vi "Edit Dialog.vi"(11 "Content":string) -> (2 "OK?":bool, 3 "String":string)   [LabVIEW 2026, in "VILab.lvlib" / "Data Item.lvclass"]
uses:
  Data Item.lvclass
panel:
  in  "Cancel":bool
  in  "OK":bool
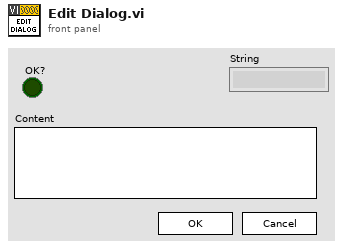
[diagram p1: front panel]
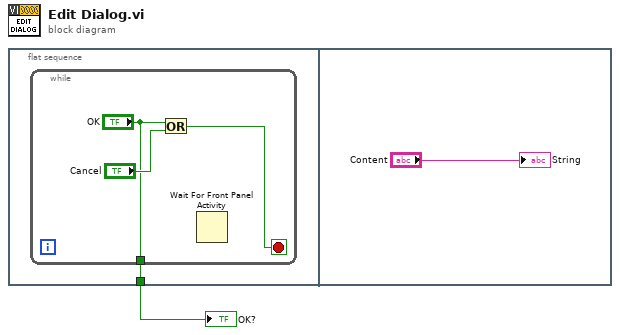
[diagram p0: block diagram]
diagram:
  n1 = flat-sequence {
    tunnel: [w2] -> w1
    frame #0 {
      n2 = while {
        tunnel: ["OK"] -> w2
        stop <- w5 stop-if-true
        n3 = Or(x="OK", y="Cancel") -> (x .or. y?=w5:bool)
        n4 = Wait For Front Panel Activity() -> ()  [unwired: 3 in, 1 out]
      }
    }
    frame #1 {
      "String" <- "Content"
    }
  }
  "OK?" <- w1
